vi "Manipulator Intake Handler v2.vi"(0 "Driver Axes":dbl[](array[numeric]), 1 "Driver Buttons":bool[](array[boolean]), 2 "Operator Axes":dbl[](array[numeric]), 3 "Operator Buttons":bool[](array[boolean]), 4 "Operator POVs":i16[](array[numeric])) -> ()   [LabVIEW 2020]
uses:
  581c7257-3437-4f1d-8e29-cfda183b7fac.vi
  manipulator/Implementation/manipulator Operations.ctl
  05bd7b36-59a4-46a9-a624-297df426cb22.vi
  Framework/Robot Global Data.vi
panel:
  in  "Operator Manual Override Scaling":dbl=0.2
  in  "Operator Manual Deadband":dbl=0.1
  in  "Driver Intake Deadband":dbl=0.2 format="%#_13g"
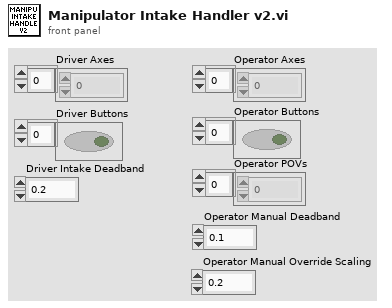
[diagram p1: front panel]
types:
  T1 = typedef "manipulator Operations.ctl" = enum16{"Reserve", "Read Current", "Immediate", "Reset Manipulator", "Grid-dy"}
  T2 = typedef "game object.ctl" = enum16{"Nothing", "Cone", "Cube"}
  T3 = cluster{"Reset Wrist":bool, "Reset Cascade":bool}
  T4 = typedef "Teleop Manipulator Commands.ctl" = enum16{"idle", "intake cone sideways", "intake cone upright", "intake cube", "score low cone", "score low cube", "score mid cone", "score mid cube", "score high cone", "score high cube"}
  T5 = typedef "Driver Controls Mode.ctl" = enum16{"Ground", "Scoring"}
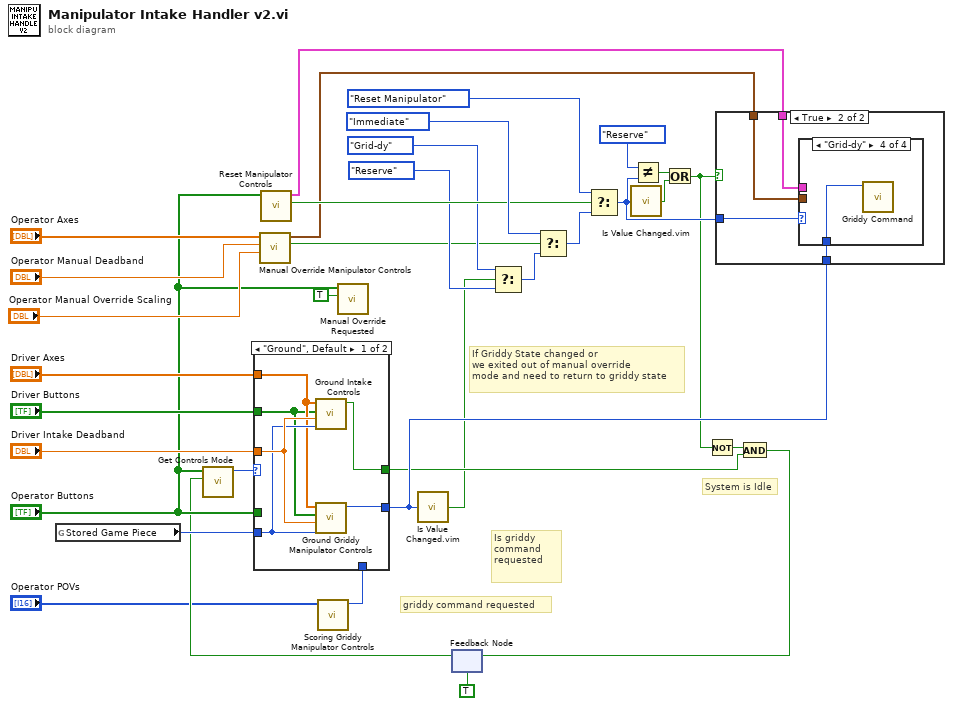
[diagram p0: block diagram]
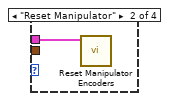
[diagram p4: hidden frame]
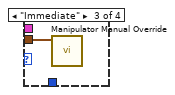
[diagram p5: hidden frame]
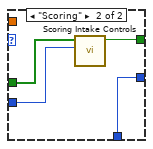
[diagram p6: hidden frame]
diagram:
  # "If Griddy State changed or\nwe exited out of manual override\nmode and need to return to griddy state"
  # "System is Idle"
  # "griddy command requested"
  # "Is griddy command requested"
  n1 = global read "Robot Global Data.vi" "Stored Game Piece"() -> (w9:T2)
  n2 = call "Manual Override Manipulator Controls.vi"("Manual Override Scaling"="Operator Manual Override Scaling", "Deadband"="Operator Manual Deadband", "Operator Axes"="Operator Axes") -> ("Manul Override Requested?"=w1:bool, "Manual Override Data"=w20:cluster{"Wrist Power":dbl, "Cascade Power":dbl})  [unwired: 7 in]
  n3 = call "Reset Manipulator Controls.vi"("Operator Buttons"="Operator Buttons") -> ("Reset Requested?"=w30:bool, "Reset Parameters"=w21:T3)  [unwired: 9 in]
  n4 = call "Scoring Griddy Manipulator Controls.vi"("Operator POVs"="Operator POVs") -> ("Griddy Data"=w3:T4)  [unwired: 10 in]
  n5 = call "Manual Override Requested.vi"("Is Idle?"=TRUE, "Operator Buttons"="Operator Buttons") -> ()  [unwired: 9 in, 1 out]
  n6 = feedback #1(TRUE) -> (w6:bool)
  n7 = call "Get Controls Mode.vi"("System is Idle?"=w6, "Operator Buttons"="Operator Buttons") -> ("Driver Controls Mode"=w34:T5)  [unwired: 9 in]
  n8 = case shown="\"Ground\", Default" w34 {
    tunnel: [w40 w41] -> w22
    tunnel: "Driver Intake Deadband" -> [w39 _]
    tunnel: w9 -> [w38 w44]
    tunnel: "Driver Axes" -> [w37 _]
    tunnel: "Driver Buttons" -> [w36 _]
    tunnel: "Operator Buttons" -> [_ w43]
    tunnel: [w35 w42] -> w12
    tunnel: w3 -> [_ w41]
    frame "Ground", Default {
      n9 = call "Ground Intake Controls.vi"(8:w38, "Deadband"=w39, "Driver Buttons"=w36, "Driver Axes"=w37) -> ("Is Idle?"=w35:bool)  [unwired: 7 in]
      n10 = call "Ground Griddy Manipulator Controls.vi"("Stored Game Piece"=w38, "Deadband"=w39, "Driver Buttons"=w36, "Driver Axes"=w37) -> ("Ground Griddy Manipulator Controls"=w40:T4)  [unwired: 7 in]
    }
    frame "Scoring" {
      n11 = call "Scoring Intake Controls.vi"(10:w44, "Operator Buttons"=w43) -> ("Is Idle?"=w42:bool)  [unwired: 9 in]
    }
  }
  n12 = call "Is Value Changed.vim"("value"=w22) -> ("changed or first call?"=w2:bool)
  n13 = Select(t=manipulator_Operations."Grid-dy" ("Operation"), s=w2, f=manipulator_Operations."Reserve" ("Operation")) -> (s? t:f=w29:T1)
  n14 = Select(t=manipulator_Operations."Immediate" ("Operation"), s=w1, f=w29) -> (s? t:f=w31:T1)
  n15 = Select(t=manipulator_Operations."Reset Manipulator" ("Operation"), s=w30, f=w31) -> (s? t:f=w23:T1)
  n16 = call "Is Value Changed.vim"("value"=w23) -> ("changed or first call?"=w26:bool)
  n17 = Not Equal?(x=manipulator_Operations."Reserve", y=w23) -> (x != y?=w25:bool)
  n18 = Or(x=w25, y=w26) -> (x .or. y?=w14:bool)
  n19 = Not(x=w14) -> (.not. x?=w13:bool)
  n20 = case shown="True" w14 {
    tunnel: w23 -> [_ w48]
    tunnel: w22 -> [_ w47]
    tunnel: w21 -> [_ w46]
    tunnel: w20 -> [_ w45]
    frame False {
    }
    frame True {
      n21 = case shown="\"Grid-dy\"" w48 {
        tunnel: w47 -> [_ _ _ w51]
        tunnel: w46 -> [_ w49 _ _]
        tunnel: w45 -> [_ _ w50 _]
        frame Default {
        }
        frame "Reset Manipulator" {
          n22 = call "Reset Manipulator Encoders.vi"("Reset Parameters"=w49) -> ()  [unwired: 10 in, 1 out]
        }
        frame "Immediate" {
          n23 = call "Manipulator Manual Override.vi"("Immediate Parameters"=w50) -> ()  [unwired: 10 in, 1 out]
        }
        frame "Grid-dy" {
          n24 = call "Griddy Command.vi"("Griddy Command"=w51) -> ()  [unwired: 10 in, 1 out]
        }
      }
    }
  }
  n25 = And(x=w13, y=w12) -> (x .and. y?=w11:bool)
  n26 = feedback-in #1(w11) -> ()
